vi "Memory.Array.Get Number of Elements.vi"(8 "error in (no error)":errorcluster, 11 "Memory.Array in":refnum<class "Memory.Array.Void.lvclass">) -> (0 "error out":errorcluster, 2 "number of elements":u64, 3 "Memory.Array out":refnum<class "Memory.Array.Void.lvclass">)   [LabVIEW 2016, in "LabVIEW Memory Manager.lvlib" / "Memory.Array.Void.lvclass"]
uses:
  Memory.Array.Void.lvclass
  Memory.Array.Void.lvclass/Memory.Array.Void.ctl
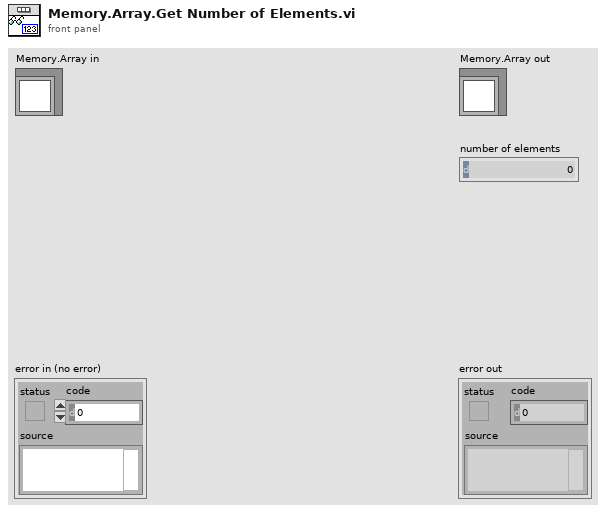
[diagram p1: front panel]
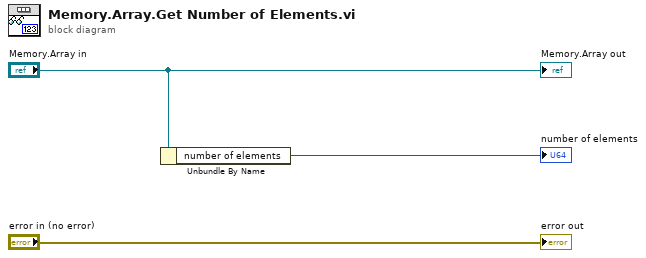
[diagram p0: block diagram]
diagram:
  n1 = Unbundle By Name("Memory.Array in") -> ("number of elements"=→"number of elements":u64)
  "error out" <- "error in (no error)"
  "Memory.Array out" <- "Memory.Array in"
